vi "DMM Read.vi"(2 "Point #":i32, 3 "Instrument Address":refnum<visa-resource-name>) -> (0 "Stop":bool, 1 "Measurement":dbl[](array[numeric]) format="%.7e")   [LabVIEW 2020]
doc: "This VI reads almost all types of multimeters and a lot of other IEEE-488 devices single reading mode. The stop boolean is always false. If no reading is obtained a single zero is returned.\nScott Hannahs, NHMFL-FSU, Nov 1993"
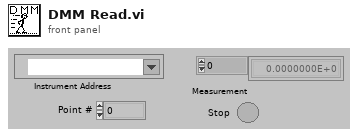
[diagram p1: front panel]
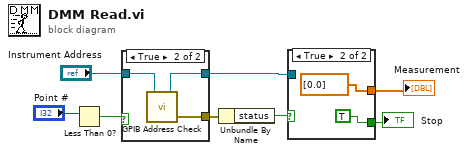
[diagram p0: block diagram]
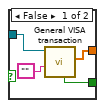
[diagram p2: hidden frame]
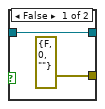
[diagram p3: hidden frame]
diagram:
  n1 = Less Than 0?(x="Point #") -> (x < 0?=w7:bool)
  n2 = case shown="True" w7 {
    tunnel: [w10 w12] -> w5
    tunnel: "Instrument Address" -> [w10 w11]
    tunnel: [errorcluster {"status"=FALSE, "code"=0, "source"=""} ("error out") w13] -> w2
    frame False {
    }
    frame True {
      n3 = call "GPIB Address Check.vi"("Instrument Address"=w11) -> ("dup VISA session"=w12:refnum<visa-resource-name>, "error out"=w13:errorcluster)  [unwired: 1 in, 1 out]
    }
  }
  n4 = Unbundle By Name(w2) -> ("status"=w1:bool)
  n5 = case shown="True" w1 {
    tunnel: w5 -> [w17 _]
    tunnel: [w15 TRUE ("Stop")] -> w4
    tunnel: [w14 dbl[] [0.0]] -> w3
    frame False {
      n6 = call "General VISA transaction.vi"("Command String"="", "VISA Session"=w17) -> ("Measurement"=w14:dbl[], "Stop"=w15:bool)  [unwired: 4 in, 4 out]
    }
    frame True {
    }
  }
  "Stop" <- w4
  "Measurement" <- w3
